vi "Read Age Wrapper - Reentrant.vi"(8 "error in (no error)":errorcluster, 11 "myClass in":refnum<class "MyClass - Reentrant.lvclass">) -> (0 "error out":errorcluster, 2 "age":dbl, 3 "myClass out":refnum<class "MyClass - Reentrant.lvclass">)   [LabVIEW 2010]
uses:
  MyClass - Reentrant.lvclass
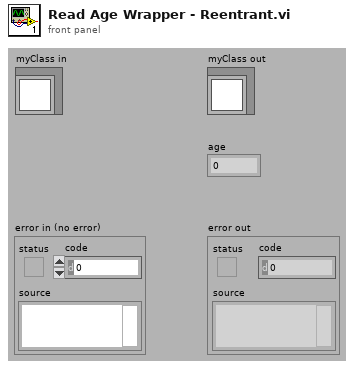
[diagram p1: front panel]
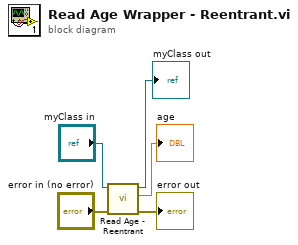
[diagram p0: block diagram]
diagram:
  n1 = call-dynamic "Read Age - Reentrant.vi"("error in (no error)"="error in (no error)", "myClass in"="myClass in") -> ("error out"=→"error out":errorcluster, "age"=→"age":dbl, "myClass out"=→"myClass out":refnum<class "MyClass - Reentrant.lvclass">)  [unwired: 7 in]
